vi "IOT表头.vi"() -> (3 "IOT信息":T1)   [LabVIEW 2017]
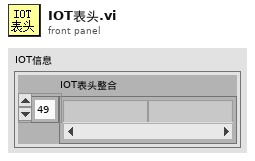
[diagram p1: front panel]
types:
  T1 = typedef "IOT信息.ctl" = cluster{"IOT表头整合":string[]}
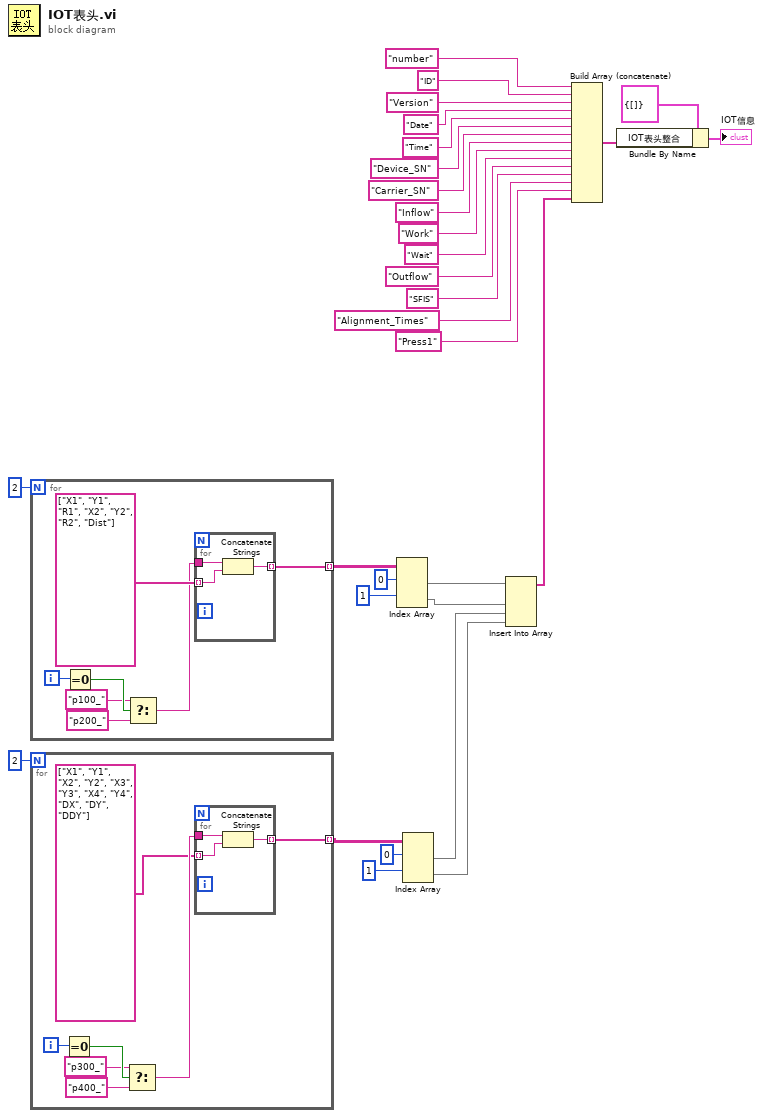
[diagram p0: block diagram]
diagram:
  n1 = for {
    N: 2 -> [_]
    tunnel: [w31] -> w11 mode=indexing
    i -> [w36]
    n2 = Equal To 0?(x=w36) -> (x = 0?=w35:bool)
    n3 = Select(t="p100_", s=w35, f="p200_") -> (s? t:f=w32:string)
    n4 = for {
      tunnel: w32 -> [w40]
      tunnel: [w39] -> w31 mode=indexing
      tunnel: string[] ["X1", "Y1", "R1", "X2", "Y2", "R2", "Dist"] ("元素") -> [w38] mode=indexing
      n5 = Concatenate Strings(w40, w38) -> (w39:string)
    }
  }
  n6 = for {
    N: 2 -> [_]
    tunnel: [w42] -> w6 mode=indexing
    i -> [w47]
    n7 = Equal To 0?(x=w47) -> (x = 0?=w46:bool)
    n8 = Select(t="p300_", s=w46, f="p400_") -> (s? t:f=w43:string)
    n9 = for {
      tunnel: w43 -> [w50]
      tunnel: [w49] -> w42 mode=indexing
      tunnel: string[] ["X1", "Y1", "X2", "Y2", "X3", "Y3", "X4", "Y4", "DX", "DY", "DDY"] ("元素") -> [w48] mode=indexing
      n10 = Concatenate Strings(w50, w48) -> (w49:string)
    }
  }
  n11 = Index Array(array=w11, index (row) #1=0 ("索引 (行)"), index (row) #2=1 ("索引 (行)")) -> (element #1=w5:string[], element #2=w4:string[])  [unwired: 2 in]
  n12 = Index Array(array=w6, index (row) #1=0 ("索引 (行)"), index (row) #2=1 ("索引 (行)")) -> (element #1=w3:string[], element #2=w2:string[])  [unwired: 2 in]
  n13 = Insert Into Array(array=w5, new element #1=w4, new element #2=w3, new element #3=w2) -> (w1:string[])  [unwired: 1 in]
  n14 = Build Array (concatenate)("number", "ID", "Version", "Date", "Time", "Device_SN", "Carrier_SN", "Inflow", "Work", "Wait", "Outflow", "SFIS", "Alignment_Times", "Press1", w1) -> (w18:string[])
  n15 = Bundle By Name(cluster=T1 {"IOT表头整合"=[]} ("IOT信息"), "IOT表头整合"=w18) -> (→"IOT信息":T1)
